vi "RT_SynthFoc_V2.vi"(0 "Ann Array Params":T1={"Synth Foc?"=FALSE, "Focal Zones"=41, "Switch T/R"=0, "Trans Geometry (mm)"={"Transducer"=0, "Geo Focus"=12.0, "a (radius)"=3.0, "# of rings"=5, "kerf space "=0.1, "Center Freq"=12.0}, "Sub Ap Excite?"=FALSE, "Full Array Scan?"=FALSE, "Xmt/Rcv"={"XMIT"=[TRUE, TRUE, TRUE, TRUE, TRUE], "RCV"=[TRUE, TRUE, TRUE, TRUE, TRUE]}, "PulseSpacing (us)"=0.0, "Xmit Ring"=0, "XMIT CHS"=0, "RCV CHS"=0, "GPU?"=FALSE, "Save TIFF?"=FALSE, "downfactor"=1, "RCV 1CH"=0} {"RCV 1CH" items=["All", "1", "2", "3", "4", "5"]; "Trans Geometry (mm)"."Transducer" items=["6D 12R 40 MHz"=0, "10D 31R 20 MHz"=1, "10D 23R 20 MHz"=2, "6D 23R 40 MHz"=3, "4.5D 10.7R 40 MHz"=4, "9D 23.5R 20 MHz"=5, "9D 25.8R 20MHz"=6, "Enter"=99]; "Switch T/R" min=1 max=5 step=1}, 2 "Pause?":bool, 3 "Motion Settings":T4={"No Motion?"=FALSE, "Motion System"=enum."NI 735x", "Motion Bd ID"=1, "Motion Profile"="SMAC1", "# Axis"=1, "Reverse Z axis?"=TRUE, "SMAC Axis"=0, "scan pair"=enum."y-(x) scan", "RT fps"=6.0, "Steps per mm"=[1000, 1000, 1000, 1000], "Motor Parameters"={"velocity ct/s"=[10000.0, 10000.0, 10000.0, 50000.0], "accel ct/s^2"=[50000.0, 50000.0, 50000.0, 200000.0]}, "One Way Scan"=FALSE, "Reverse One Way Scan"=FALSE, "Global Position (mm)"=[], "Plane"=0, "Distance between\nscan lines (um)"=0.0, "Distance between\nscan planes (um)"=0.0, "number of scan planes"=1, "Total steps in line"=0, "Xtra plane\ndistance  (um)"=100, "Xtra planes "=1, "Add Axis"=FALSE, "overshoot cts"=200, "BKPT Shift"=0, "Scan Start Time (ms)"=0, "ESP VISA"="GPIB::1::INSTR", "3rd Axis"=1, "GL Ref Out"=refnum, "Galil Address"=""} {"3rd Axis" items=["x", "y", "z", "w"]; "Xtra planes" min=1; "Xtra plane\ndistance  (um)" min=0; "Distance between\nscan planes (um)" format="%.2f"; "Distance between\nscan lines (um)" format="%.2f"; "SMAC Axis" items=["None"=0, "Axis 1"=1, "Axis 2"=2, "Axis 3"=3, "Axis 4"=4, "Axis 5"=5, "Axis 6"=6, "Axis 7"=7, "Axis 8"=8, "Vector Space 1"=17, "Vector Space 2"=18, "Vector Space 3"=19, "Vector Space 4"=20]; "Motion Bd ID" min=1 max=32 step=1}, 4 "Scan Axis":i32, 7 "Digitizer Settings":T8={"Digitizer delay (us) "=0.0, "rf points per line"=2048, "lines per plane"=128, "Samp Rate (Hz)"=100000000.0, "Additional dig delay (us)"=0.0, "Voltage Scale"=0.4, "Pre-Looks"=0, "Offset delay (us)"=0.0, "bits A/D"=8, "Avg Num"=1, "DigTimeOut"=5.0, "Rel Dig Delay"=0.0, "Dig Ch"=0, "LeCroyCluster"={"LeCroy Channels"=[TRUE, FALSE, FALSE, FALSE], "LC read pt offset"=0.0, "Sweep Avg"=FALSE}, "Main Digitizer"=enum."NI Digitizer", "Dig Config"=enum."Single channel", "Digitizer ID Cluster"={"Acqiris/Alazar/SP ID"=[], "NI Instr Handles"=[], "LeCroy VISA"="", "GaGe Handle"={"Handle"=0, "Sample size"=0, "Resolution"=0, "Offset"=0, "Channels"=0, "Boards"=0}, "ATS Ref"="ATS9350", "Acqiris Address"=["PCI::INSTR0"], "ADQRef"=refnum, "adq_cu_ptr"=refnum}, "Trigger Settings"={"Trig Source"=1, "Trig Coupling"=0, "Trig Slope"=0, "Level (mV)"=1500.0}, "Bulk Acq"=FALSE, "Bulk Start Indexes"=[], "Data Ref RF"=refnum, "NI ID/Channel"=[], "Total Dig CH"=1, "Xtra Ann Trig delay (us)"=10.0, "Fix Z Delay?"=FALSE, "One Way Transmission?"=FALSE, "Data Ref Log"=refnum} {"Trigger Settings"."Trig Slope" items=["Positive", "Negative"]; "Trigger Settings"."Level (mV)" format="%.2f"; "Trigger Settings"."Trig Coupling" items=["DC 1 MOhm", "AC 1 MOhm", "DC 50 Ohm", "AC 50 Ohm"]; "Trigger Settings"."Trig Source" items=["Chan 1", "External"]; "Rel Dig Delay" format="%.2f"; "DigTimeOut" format="%.2f"; "Avg Num" min=1; "Offset delay (us)" format="%.2f"; "Additional dig delay (us)" format="%.2f"; "Digitizer delay (us)" format="%.2f"}, 8 "Filter":T12, 9 "Qs and Notis":T13, 11 "Raw Name":string="raw") -> (16 "Bd ID Out":u8, 19 "error out":errorcluster)   [LabVIEW 2022 SP3]
uses:
  <vilib>/picture/picture.llb/imagedata.ctl
  ScanningControl/Digitizers/-DigitizerRoutines/DigitizerSettings.ctl
  ScanningControl/Digitizers/-DigitizerRoutines/Digitizer.ctl
  ScanningControl/Digitizers/-DigitizerRoutines/DigConfig.ctl
  ScanningControl/Digitizers/-DigitizerRoutines/DigitizerID.ctl
  C:/Windows/System32/ADQAPI_dotNet_helper.dll
  Windows/System32/ADQAPI_dotNet_helper.dll
  ScanningControl/Motion Controllers/NI_controller/-NI_MotionRoutines/MotionParameters.ctl
  ScanningControl/Motion Controllers/NI_controller/-NI_MotionRoutines/MotionSys.ctl
  ScanningControl/Motion Controllers/-MotionRoutines/ScanAxis.ctl
  ScanningControl/Motion Controllers/-MotionRoutines/3rdAxis.ctl
  Annular Array/-AnnularRoutines/AnnularArray.ctl
  Annular Array/-AnnularRoutines/TransGeometry.ctl
  Annular Array/-AnnularRoutines/ArrayGeometry.ctl
  ScanningControl/Motion Controllers/Galil/Command Menu.ctl
  <vilib>/DAQmx/write.llb/DAQmx Write (Digital Bool 1Line 1Point).vi
  <instrlib>/niScope/Acquire/niScope Get Scaling Coefficients.vi
  ScanningControl/Motion Controllers/-MotionRoutines/MotionGlobals.vi
  <vilib>/DAQmx/miscellaneous.llb/DAQmx Fill In Error Info.vi
  <instrlib>/niScope/Acquire/Fetch/niScope Multi Fetch Binary 8.vi
  <vilib>/Motion/FlexMotion/FunctionsVIs/Trajectory.llb/Load Acceleration/Deceleration.flx
  <vilib>/Motion/FlexMotion/CustomControls/CustomControls.llb/Program.flx
  <instrlib>/LeCroy Wave Series/LeCroy Wave Series.lvlib
  <vilib>/Motion/FlexMotion/FunctionsVIs/Trajectory.llb/Wait for Move Complete (8 axes).flx
panel:
  in  "Round to ROC?":bool
  in  "One Way Receive":bool
  # "1-D and 2-D B scan settings"
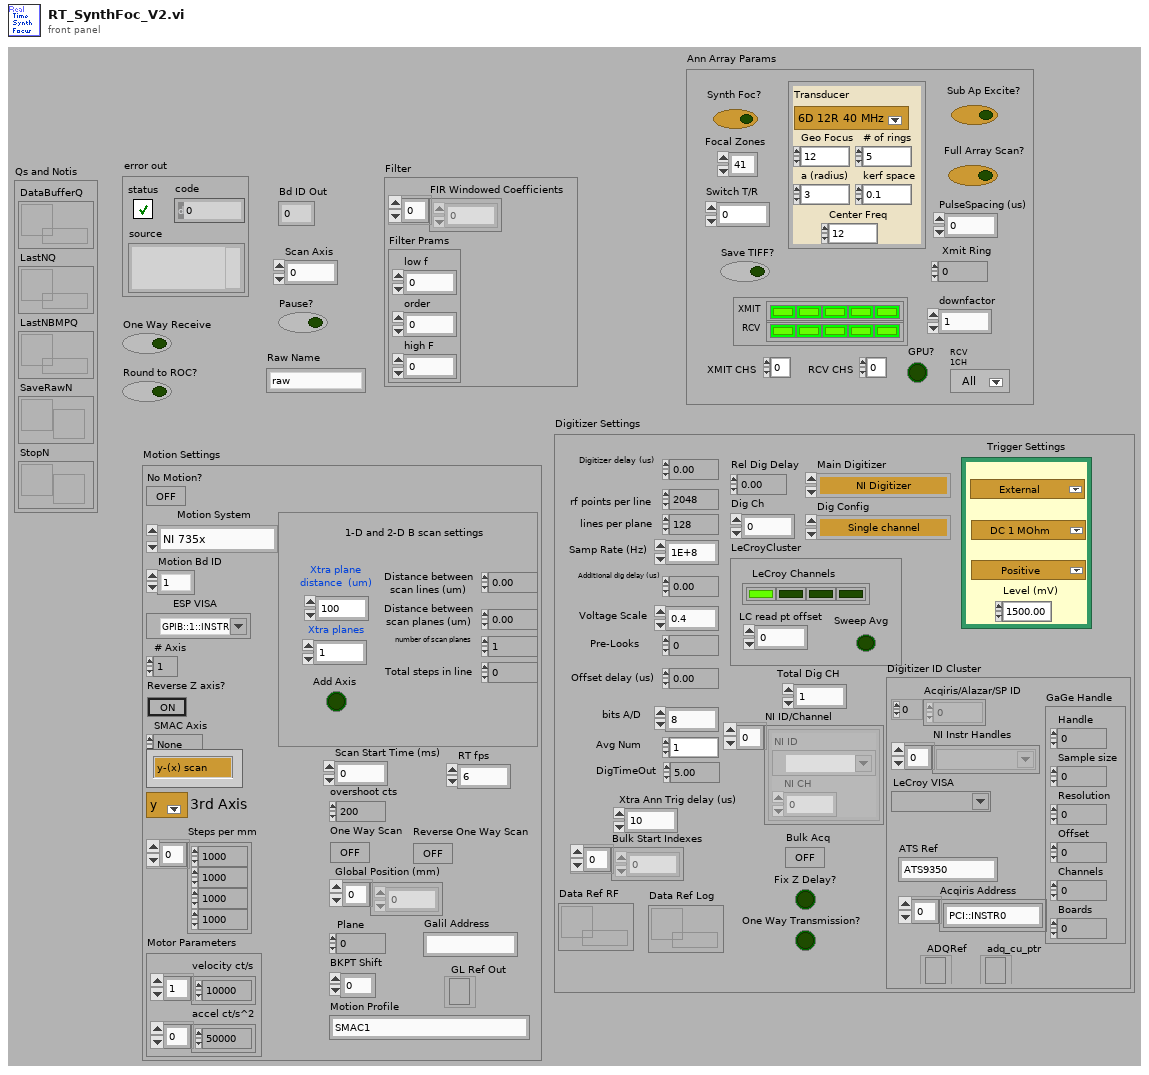
[diagram p1: front panel]
types:
  T1 = typedef "AnnularArray.ctl" = cluster{"Synth Foc?":bool, "Focal Zones":i16, "Switch T/R":i16, "Trans Geometry (mm)":T2, "Sub Ap Excite?":bool, "Full Array Scan?":bool, "Xmt/Rcv":cluster{"XMIT":bool[], "RCV":bool[]}, "PulseSpacing (us)":sgl, "Xmit Ring":i32, "XMIT CHS":u8, "RCV CHS":u8, "GPU?":bool, "Save TIFF?":bool, "downfactor":i32, "RCV 1CH":u16}
  T2 = typedef "TransGeometry.ctl" = cluster{"Transducer":T3, "Geo Focus":dbl, "a (radius)":dbl, "# of rings":i32, "kerf space ":dbl, "Center Freq":dbl}
  T3 = typedef "ArrayGeometry.ctl" = u16
  T4 = typedef "MotionParameters.ctl" = cluster{"No Motion?":bool, "Motion System":T5, "Motion Bd ID":u8, "Motion Profile":string, "# Axis":i8, "Reverse Z axis?":bool, "SMAC Axis":u16, "scan pair":T6, "RT fps":sgl, "Steps per mm":i32[], "Motor Parameters":cluster{"velocity ct/s":dbl[], "accel ct/s^2":dbl[]}, "One Way Scan":bool, "Reverse One Way Scan":bool, "Global Position (mm)":dbl[], "Plane":i32, "Distance between\nscan lines (um)":sgl, "Distance between\nscan planes (um)":sgl, "number of scan planes":i32, "Total steps in line":i32, "Xtra plane\ndistance  (um)":i32, "Xtra planes ":i32, "Add Axis":bool, "overshoot cts":i32, "BKPT Shift":i32, "Scan Start Time (ms)":u32, "ESP VISA":refnum<visa-resource-name>, "3rd Axis":T7, "GL Ref Out":refnum<k7>, "Galil Address":string}
  T5 = typedef "MotionSys.ctl" = enum16{"MM3000", "NI 735x", "Newport ESP", "No Motion Card", "Galil"}
  T6 = typedef "ScanAxis.ctl" = enum16{"y-(x) scan", "x-(y) scan", "z-(x) scan", "z-(y) scan", "y-(z) scan", "x-(z) scan", "w-(x) scan", "w-(y) scan", "w-(z) scan", "x-(w) scan", "y-(w) scan", "z-(w) scan"}
  T7 = typedef "3rdAxis.ctl" = u16
  T8 = typedef "DigitizerSettings.ctl" = cluster{"Digitizer delay (us) ":dbl, "rf points per line":i32, "lines per plane":i32, "Samp Rate (Hz)":dbl, "Additional dig delay (us)":dbl, "Voltage Scale":dbl, "Pre-Looks":i32, "Offset delay (us)":dbl, "bits A/D":i8, "Avg Num":i32, "DigTimeOut":sgl, "Rel Dig Delay":sgl, "Dig Ch":i32, "LeCroyCluster":cluster{"LeCroy Channels":bool[], "LC read pt offset":dbl, "Sweep Avg":bool}, "Main Digitizer":T9, "Dig Config":T10, "Digitizer ID Cluster":T11, "Trigger Settings":cluster{"Trig Source":u16, "Trig Coupling":u16, "Trig Slope":u16, "Level (mV)":dbl}, "Bulk Acq":bool, "Bulk Start Indexes":i32[], "Data Ref RF":refnum<data-value>, "NI ID/Channel":cluster{"NI ID":refnum<k15>, "NI CH":i32}[], "Total Dig CH":i32, "Xtra Ann Trig delay (us)":dbl, "Fix Z Delay?":bool, "One Way Transmission?":bool, "Data Ref Log":refnum<data-value>}
  T9 = typedef "Digitizer.ctl" = enum16{"Acqiris Digitizer", "NI Digitizer", "LeCroy", "GaGe", "AlazarTech", "No Digitizer", "Teledyne"}
  T10 = typedef "DigConfig.ctl" = enum16{"Single channel", "2 Chans w/ 2 Acqiris", "2 Chans w/ 1 Acqiris", "5-CH Pulser New", "5-CH pulser w/ ann array", "5-pass style ann array", "Empty"}
  T11 = typedef "DigitizerID.ctl" = cluster{"Acqiris/Alazar/SP ID":u32[], "NI Instr Handles":refnum<k15>[], "LeCroy VISA":refnum<visa-resource-name>, "GaGe Handle":cluster{"Handle":u32, "Sample size":u32, "Resolution":i32, "Offset":i32, "Channels":u32, "Boards":u32}, "ATS Ref":string, "Acqiris Address":string[], "ADQRef":refnum<k24>, "adq_cu_ptr":refnum<k24>}
  T12 = cluster{"FIR Windowed Coefficients":dbl[], "Filter Prams":cluster{"low f":i32, "order":i32, "high F":i32}}
  T13 = cluster{"DataBufferQ":refnum<queue>, "LastNQ":refnum<queue>, "LastNBMPQ":refnum<queue>, "SaveRawN":refnum<notifier>, "StopN":refnum<notifier>}
  T14 = cluster{"offset":dbl, "gain":dbl, "reserved 1":dbl, "reserved 2":dbl}[]
  T15 = cluster{"offset":dbl, "gain":dbl, "reserved 1":dbl, "reserved 2":dbl}
  T16 = cluster{sgl, "Gain [dB]  ":sgl, "Atten (dB)":sgl}
  T17 = typedef "location.ctl" = enum16{"Automatic", "WCM Main", "Hawaii", "Columbia MM3000", "Columbia  NI System", "NYU", "RRI 2", "UHI Allen", "CUMC RT", "Chiba", "Stony Brook", "WCM Microscopy", "WCM Aeoretch", "WCM Optics Lab", "WCM Main 2Axis", "WCM Rotation", "WCM SAM SMAC", "SERI GP"}
  T18 = typedef "Command Menu.ctl" = enum16{"CommandPassThrough", "Abort Motion", "Define Pos", "Velocity", "Acceleration", "Deceleration", "Position Rel", "Postion Abs", "Begin Move", "After Move", "Home", "KI", "KD", "KP", "IL", "Config I/O", "Set Bit", "Clear Bit", "Motor Off", "Moto On", "Status", "Execute", "Halt Execute", "HX Status", "Tell Velocity", "Check Motion", "BreakPoint", "Tell Position", "Current Code Line", "Tell Switches", "OC Force On", "OC Off", "Pos Soft Limit", "Rev Soft Limit"}
  T19 = cluster{"gain":dbl, "wfm":i16[][], bool, "max queue size (-1, unlimited)":i32, bool}
  T20 = typedef "Program.flx" = u8
  T21 = cluster{"Y Scale Offset":dbl, "Y Scale Multi":dbl, "X Scale Offset":dbl, "X Scale Multi":dbl, "Gate Distance":dbl}
  T22 = cluster{"ZoneStart":sgl[], "ZoneShift":sgl[], "ZoneLength":sgl[]}
  T23 = cluster{"data value reference":refnum<data-value>, "bytes to transfer":u32, "rf pts actual":u32}
  T24 = cluster{"gain":dbl, bool, i16[][], "Sat Pts":i32, bool}
  T25 = cluster{"actualSamples":i32, "absoluteInitialX":dbl, "relativeInitialX":dbl, "xIncrement":dbl, "offset":dbl, "gain":dbl, "reserved1":dbl, "reserved2":dbl}[]
  T26 = cluster{"actualSamples":i32, "absoluteInitialX":dbl, "relativeInitialX":dbl, "xIncrement":dbl, "offset":dbl, "gain":dbl, "reserved1":dbl, "reserved2":dbl}
  T27 = cluster{"gain":dbl, "wfm":i16[][], "Reverse?":bool, i32, "status":bool}
  T28 = cluster{"Voltage Scale":dbl, i16[][], "Reverse?":bool, i32, bool}
  T29 = cluster{"Raw VGain (scale)":dbl, i16[][], "Reverse?":bool, i32, "x = y?":bool}
  T30 = typedef "Bd Id Out" = u8
  T31 = typedef "Resource Out (Enum).flx" = u16
  T32 = typedef "GL Axis Control.ctl" = u16
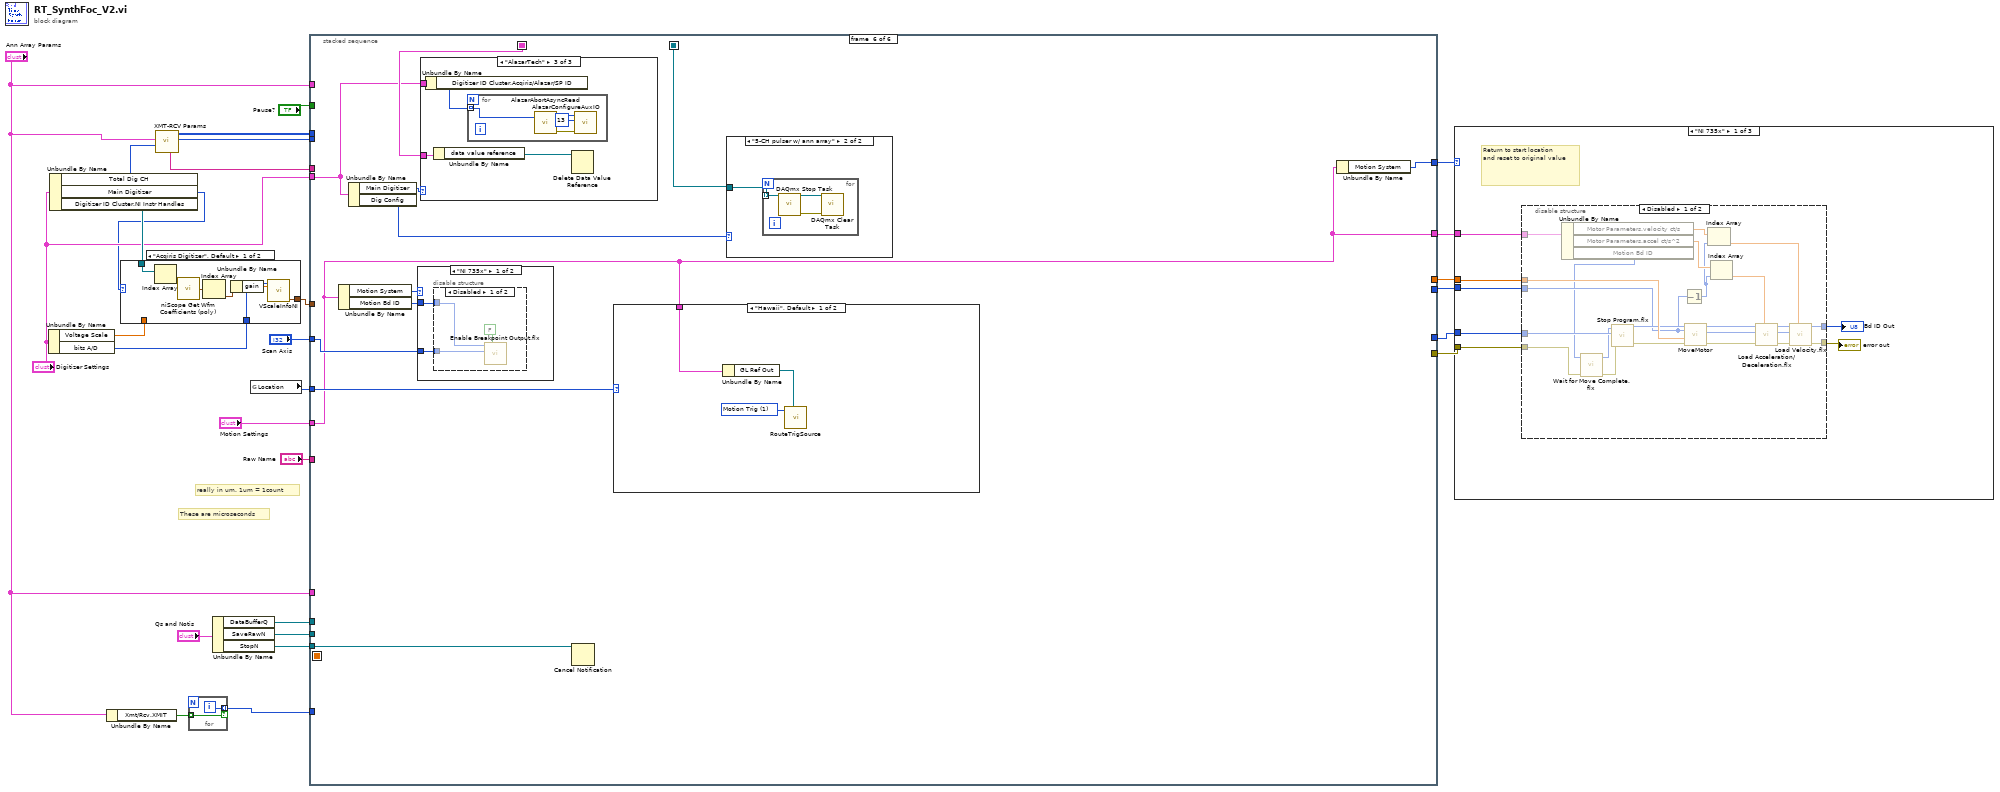
[diagram p0: block diagram]
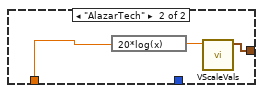
[diagram p2: hidden frame]
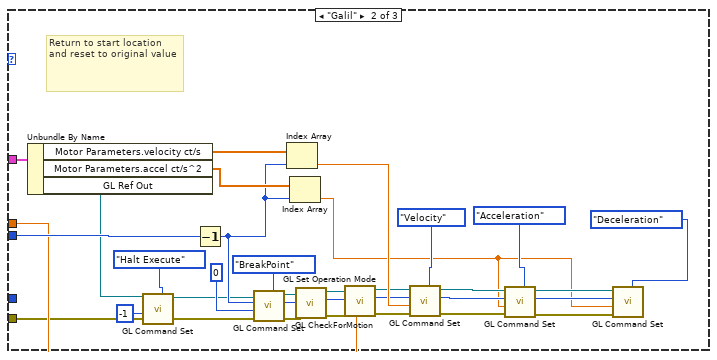
[diagram p4: hidden frame]
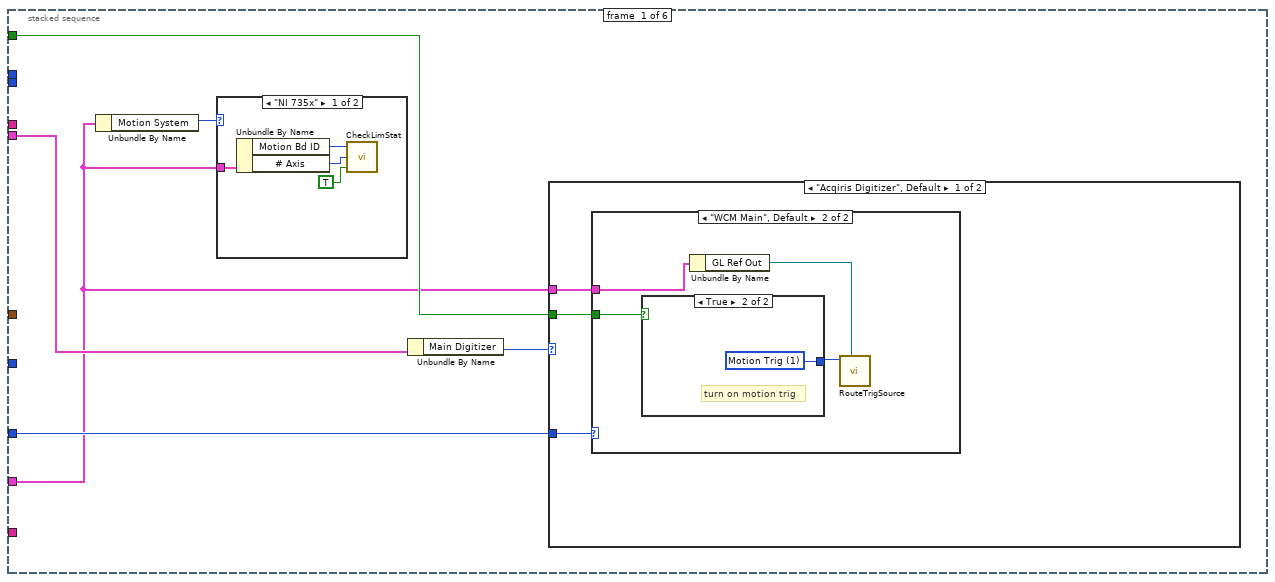
[diagram p6: hidden frame]
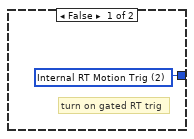
[diagram p8: hidden frame]
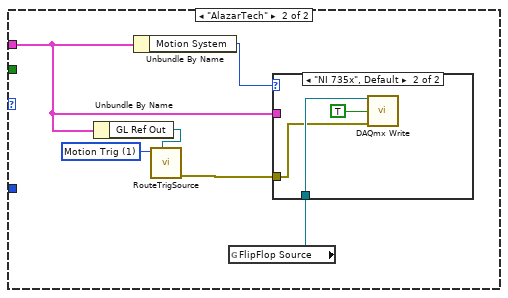
[diagram p9: hidden frame]
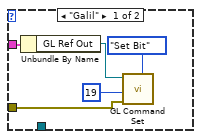
[diagram p10: hidden frame]
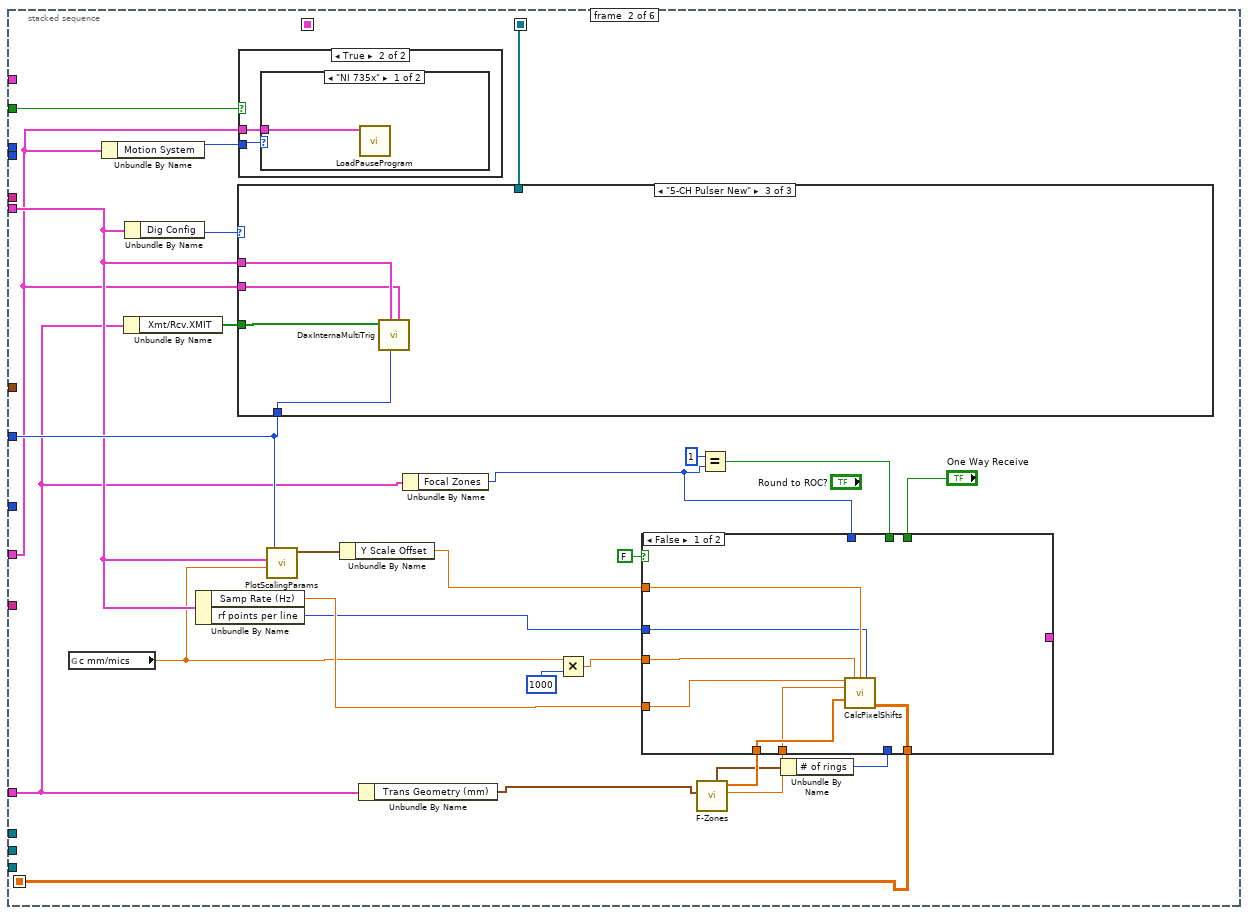
[diagram p12: hidden frame]
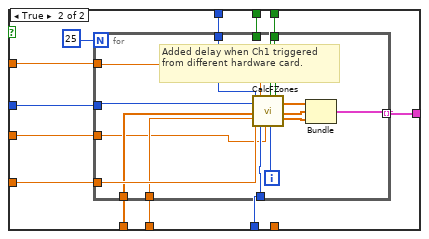
[diagram p13: hidden frame]
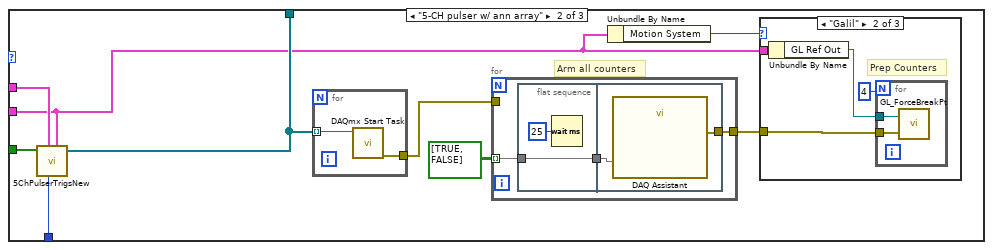
[diagram p15: hidden frame]
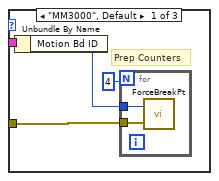
[diagram p16: hidden frame]
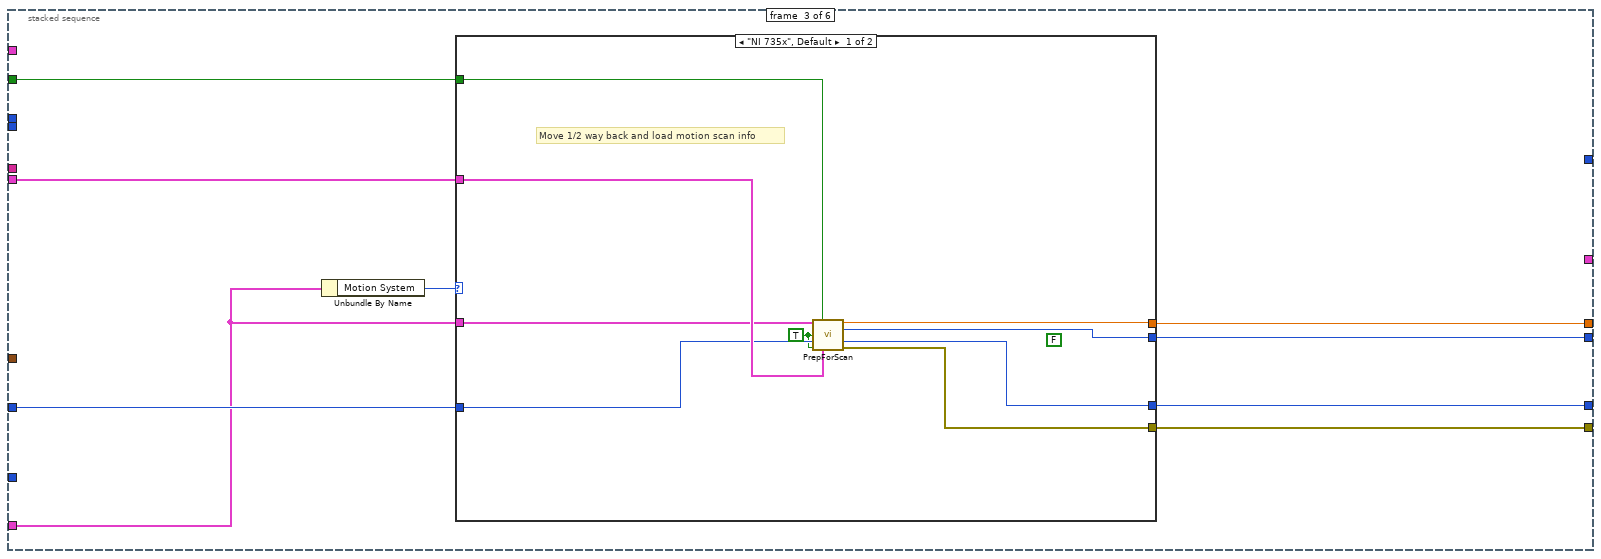
[diagram p20: hidden frame]
diagram:
  # "These are microseconds"
  # "really in um. 1um = 1count"
  n1 = Unbundle By Name("Digitizer Settings") -> ("Voltage Scale"=w13:dbl, "bits A/D"=w12:i8)
  n2 = Unbundle By Name("Digitizer Settings") -> ("Total Dig CH"=w4:i32, "Main Digitizer"=w10:T9, "Digitizer ID Cluster.NI Instr Handles"=w14:refnum<k15>[])
  n3 = Unbundle By Name("Ann Array Params") -> ("Xmt/Rcv.XMIT"=w3:bool[])
  n4 = case shown="\"Acqiris Digitizer\", Default" w10 {
    tunnel: [w31 w37] -> w17
    tunnel: w14 -> [w30 _]
    tunnel: w12 -> [w29 _]
    tunnel: w13 -> [_ w36]
    frame "Acqiris Digitizer", Default {
      n5 = Index Array(array=w30) -> (element=w33:refnum<k15>)  [unwired: 1 in]
      n6 = call-poly <instrlib>:"niScope Get Wfm Coefficients (poly).vi"("instrument handle"=w33) -> ("coefficient info"=w34:T14)  [unwired: 12 in, 2 out]
      n7 = Index Array(array=w34) -> (element=w35:T15)  [unwired: 1 in]
      n8 = Unbundle By Name(w35) -> ("gain"=w32:dbl)
      n9 = call "VScaleInfoNI.vi"("A/D bits"=w29, "gain"=w32) -> ("Voltage Scale"=w31:T16)  [unwired: 5 in, 3 out]
    }
    frame "AlazarTech" {
      n10 = expression code="20*log(x)"(w36) -> (w38:dbl)
      n11 = call "VScaleVals.vi"("Full Scale"=w38) -> ("Voltage Scale"=w37:T16)  [unwired: 8 in, 2 out]
    }
  }
  n12 = call "XMT-RCV Params.vi"("Dig Channels"=w4, "Ann Array Params"="Ann Array Params") -> ("# XMIT"=w16:i16, "Recip Table"=w15:i16[][], "T/R String"=w9:string)  [unwired: 4 in, 3 out]
  n13 = for {
    tunnel: w3 -> [w39] mode=indexing
    tunnel: [w40] -> w1 mode=indexing if=w39
    i -> [w40]
  }
  n14 = Unbundle By Name("Qs and Notis") -> ("DataBufferQ"=w22:refnum<queue>, "SaveRawN"=w21:refnum<notifier>, "StopN"=w23:refnum<notifier>)
  n15 = global read "MotionGlobals.vi" "Location"() -> (w18:T17)
  n16 = stacked-sequence {
    seq-local: [_ w74 _ _ _ _] -> [_ _ _ _ w248 _]
    seq-local: [_ w98 _ _ _ _] -> [_ _ _ _ _ w679]
    seq-local: [_ _ _ w195 _ _] -> [_ _ _ _ w260 w675]
    tunnel: [_ _ w180 _ _ _] -> w26
    tunnel: [_ _ w179 _ _ _] -> w27
    tunnel: [_ _ w176 _ _ _] -> w25
    tunnel: [_ _ w178 _ _ _] -> w28
    tunnel: "Scan Axis" -> [_ w91 w177 _ _ w676]
    tunnel: w23 -> [_ _ _ _ w289 w677]
    tunnel: w22 -> [_ _ _ _ w274 _]
    tunnel: w18 -> [w46 _ _ _ _ w678]
    tunnel: "Pause?" -> [w45 w99 w175 w190 w286 _]
    tunnel: w21 -> [_ _ _ _ w285 _]
    tunnel: "Raw Name" -> [_ _ _ _ w284 _]
    tunnel: w17 -> [_ _ _ _ w282 _]
    tunnel: w16 -> [_ _ _ w197 w280 _]
    tunnel: w15 -> [_ _ _ _ w255 _]
    tunnel: w9 -> [_ _ _ _ w279 _]
    tunnel: "Digitizer Settings" -> [w43 w87 w174 w192 w250 w674]
    tunnel: "Motion Settings" -> [w41 w79 w173 _ w265 w668]
    tunnel: [_ _ _ _ _ w669] -> w8
    tunnel: [_ _ _ _ _ w668] -> w7
    tunnel: "Ann Array Params" -> [_ w81 _ _ w252 _]
    tunnel: "Ann Array Params" -> [_ _ _ _ w254 _]
    tunnel: w1 -> [_ _ _ _ w249 _]
    frame #0 {
      n17 = Unbundle By Name(w41) -> ("Motion System"=w42:T5)
      n18 = case shown="\"NI 735x\"" w42 {
        tunnel: w41 -> [w73 _]
        frame "NI 735x" {
          n19 = Unbundle By Name(w73) -> ("Motion Bd ID"=w72:u8, "# Axis"=w71:i8)
          n20 = call "CheckLimStat.vi"("Always Warn?"=TRUE, "# Axis"=w71, "Motion Board ID"=w72) -> ()  [unwired: 3 in]
        }
        frame "Newport ESP", "No Motion Card", Default {
        }
      }
      n21 = Unbundle By Name(w43) -> ("Main Digitizer"=w44:T9)
      n22 = case shown="\"Acqiris Digitizer\", Default" w44 {
        tunnel: w46 -> [w49 _]
        tunnel: w45 -> [w48 _]
        tunnel: w41 -> [w47 w57]
        frame "Acqiris Digitizer", Default {
          n23 = case shown="\"WCM Main\", Default" w49 {
            tunnel: w48 -> [_ w53]
            tunnel: w47 -> [_ w51]
            frame "UHI Allen", "CUMC RT" {
            }
            frame "WCM Main", Default {
              n24 = case shown="True" w53 {
                tunnel: [w54 w55] -> w52
                frame False {
                  w54 = u16 2 items=["Function Gen Input", "Motion Trig", "Internal RT Motion Trig", "Internal CTR 1 Output"] ("Trig Source")
                  # "turn on gated RT trig"
                }
                frame True {
                  w55 = u16 1 items=["Function Gen Input", "Motion Trig", "Internal RT Motion Trig", "Internal CTR 1 Output"] ("Trig Source")
                  # "turn on motion trig"
                }
              }
              n25 = Unbundle By Name(w51) -> ("GL Ref Out"=w50:refnum<k7>)
              n26 = call "RouteTrigSource.vi"("Galil.IGalil"=w50, "Trig Source"=w52) -> ()  [unwired: 9 in, 1 out]
            }
          }
        }
        frame "AlazarTech" {
          w61 = u16 1 items=["Function Gen Input", "Motion Trig", "Internal RT Motion Trig", "Internal CTR 1 Output"] ("Trig Source")
          n27 = Unbundle By Name(w57) -> ("GL Ref Out"=w56:refnum<k7>)
          n28 = Unbundle By Name(w57) -> ("Motion System"=w59:T5)
          n29 = call "RouteTrigSource.vi"("Galil.IGalil"=w56, "Trig Source"=w61) -> ("error out"=w58:errorcluster)  [unwired: 9 in]
          n30 = global read "MotionGlobals.vi" "FlipFlop Source"() -> (w60:refnum<k21>)
          n31 = case shown="\"NI 735x\", Default" w59 {
            tunnel: w60 -> [_ w68]
            tunnel: w57 -> [w63 _]
            tunnel: w58 -> [w62 w67]
            frame "Galil" {
              n32 = Unbundle By Name(w63) -> ("GL Ref Out"=w66:refnum<k7>)
              n33 = call "GL Command Set.vi"("Command"=Command_Menu."Set Bit", "error in (no error)"=w62, "Value"=19, "Galil.IGalil"=w66) -> ()  [unwired: 3 in, 5 out]
            }
            frame "NI 735x", Default {
              n34 = call-poly <vilib>:"DAQmx Write.vi"("task/channels in"=w68, "data"=TRUE ("stop (T)"), "error in"=w67) -> ()  [unwired: 10 in, 3 out]
            }
          }
        }
      }
    }
    frame #1 {
      n35 = global read "MotionGlobals.vi" "c mm/mics"() -> (w77:sgl)
      n36 = Unbundle By Name(w79) -> ("Motion System"=w86:T5)
      n37 = Unbundle By Name(w81) -> ("Xmt/Rcv.XMIT"=w82:bool[])
      n38 = Unbundle By Name(w87) -> ("Dig Config"=w88:T10)
      n39 = Unbundle By Name(w87) -> ("Samp Rate (Hz)"=w93:dbl, "rf points per line"=w92:i32)
      n40 = case shown="\"5-CH Pulser New\"" w88 {
        tunnel: w91 -> [_ w143 w165]
        tunnel: [_ w142 _] -> w98
        tunnel: w82 -> [_ w138 w166]
        tunnel: w87 -> [_ w137 w168]
        tunnel: w79 -> [_ w135 w167]
        frame "Single channel", Default {
        }
        frame "5-CH pulser w/ ann array" {
          # "Arm all counters"
          n41 = call "5ChPulserTrigsNew.vi"("Motion Settings"=w135, "Digitizer Settings"=w137, "XMIT"=w138, "Axis"=w143) -> ("5CH Pulser Tasks"=w142:refnum<k21>[])  [unwired: 5 in, 1 out]
          n42 = for {
            tunnel: w142 -> [w157] mode=indexing
            tunnel: [w156] -> w140
            n43 = call <vilib>:"DAQmx Start Task.vi"("task/channels in"=w157) -> ("error out"=w156:errorcluster)  [unwired: 1 in, 13 out]
          }
          n44 = for {
            tunnel: bool[][] [[TRUE], [FALSE]] ("data") -> [w159] mode=indexing
            tunnel: w140 -> [_]
            tunnel: [w158] -> w139
            n45 = flat-sequence {
              tunnel: w159 -> [w162]
              tunnel: [w162] -> w160
              tunnel: w160 -> [w164]
              tunnel: [w163] -> w158
              frame #0 {
                n46 = Wait (ms)(milliseconds to wait=u32 25) -> ()  [unwired: 1 out]
              }
              frame #1 {
                n47 = call "DAQ Assistant"("data"=w164) -> ("error out"=w163:errorcluster)  [unwired: 17 in, 1 out]
              }
            }
          }
          n48 = Unbundle By Name(w135) -> ("Motion System"=w136:T5)
          n49 = case shown="\"Galil\"" w136 {
            tunnel: w139 -> [w146 w152 _]
            tunnel: w135 -> [w145 w150 _]
            frame "MM3000", Default {
              # "Prep Counters"
              n50 = Unbundle By Name(w145) -> ("Motion Bd ID"=w144:u8)
              n51 = for {
                N: 4 -> [_]
                tunnel: w144 -> [w149]
                tunnel: w146 -> [w148]
                n52 = call "ForceBreakPt.vi"("error in"=w148, "Bd ID in"=w149) -> ()  [unwired: 2 out]
              }
            }
            frame "Galil" {
              # "Prep Counters"
              n53 = Unbundle By Name(w150) -> ("GL Ref Out"=w151:refnum<k7>)
              n54 = for {
                N: 4 -> [_]
                tunnel: w151 -> [w155]
                tunnel: w152 -> [w154]
                n55 = call "GL_ForceBreakPt.vi"("error in"=w154, "GL Ref Out"=w155) -> ()  [unwired: 2 out]
              }
            }
            frame "No Motion Card" {
            }
          }
        }
        frame "5-CH Pulser New" {
          n56 = call "DaxInternaMultiTrig.vi"("Motion Settings"=w167, "Digitizer Settings"=w168, "XMIT"=w166, "Axis"=w165) -> ()  [unwired: 6 in, 1 out]
        }
      }
      n57 = case shown="True" w99 {
        tunnel: w86 -> [_ w170]
        tunnel: w79 -> [_ w169]
        frame False {
        }
        frame True {
          n58 = case shown="\"NI 735x\"" w170 {
            tunnel: w169 -> [w171 _]
            frame "NI 735x" {
              n59 = call "LoadPauseProgram.vi"("Motion Settings"=w171) -> ()  [unwired: 10 in, 1 out]
            }
            frame "No Motion Card", Default {
            }
          }
        }
      }
      n60 = call "PlotScalingParams.vi"("c mm/mics"=w77, "Digitizer Settings"=w87, "Scan Axis"=w91) -> ("Cluster"=w90:T21)  [unwired: 6 in, 2 out]
      n61 = Unbundle By Name(w90) -> ("Y Scale Offset"=w89:dbl)
      n62 = Unbundle By Name(w81) -> ("Trans Geometry (mm)"=w83:T2)
      n63 = Unbundle By Name(w81) -> ("Focal Zones"=w80:i16)
      n64 = Multiply(x=w77, y=1000) -> (x*y=w76:sgl)
      n65 = call "F-Zones.vi"("Trans Geometry (mm)"=w83) -> ("ROC (m)"=w96:dbl, "annuli rad (m)"=w97:dbl[], "Trans Geometry (mm) out"=w85:T2)  [unwired: 7 in, 1 out]
      n66 = Equal?(x=i16 1, y=w80) -> (x = y?=w94:bool)
      n67 = Unbundle By Name(w85) -> ("# of rings"=w84:i32)
      n68 = case shown="False" FALSE {
        tunnel: "One Way Receive" -> [_ w119]
        tunnel: w97 -> [w106 w117]
        tunnel: w96 -> [w105 w116]
        tunnel: [_ w115] -> _
        tunnel: w94 -> [_ w114]
        tunnel: w93 -> [w107 w113]
        tunnel: w92 -> [w102 w112]
        tunnel: w89 -> [w103 w111]
        tunnel: w76 -> [w104 w110]
        tunnel: w84 -> [_ w109]
        tunnel: w80 -> [_ w108]
        tunnel: [w101 _] -> w74
        frame False {
          n69 = call "CalcPixelShifts.vi"("Sampling Rate (Hz)"=w107, "c (m/s)"=w104, "delay (mm)"=w103, "rf pts"=w102, "ROC (m)"=w105, "Radii (m)"=w106) -> ("InterpIndex"=w101:sgl[][])  [unwired: 9 in]
        }
        frame True {
          n70 = for {
            N: 25 -> [_]
            tunnel: w112 -> [w134]
            tunnel: w110 -> [w120]
            tunnel: w113 -> [w129]
            tunnel: w111 -> [w122]
            tunnel: w119 -> [w133]
            tunnel: w114 -> [w132]
            tunnel: [w130] -> w115 mode=indexing
            tunnel: w117 -> [w126]
            tunnel: w116 -> [w125]
            tunnel: w108 -> [w123]
            tunnel: w109 -> [w121]
            i -> [w124]
            # "Added delay when Ch1 triggered from different hardware card."
            n71 = call "CalcFZones.vi"("F- zones"=w123, "# rf points per line"=w134, "Radii (m)"=w126, "ROC (m)"=w125, "Sampling Rate"=w129, "delay (mm)"=w122, "# Elements"=w121, "c (m/s)"=w120, "Round to ROC?"=w132, "File index number"=w124, "One Way Receive"=w133) -> ("ZoneStart"=w128:sgl[], "ZoneShift"=w127:sgl[], "ZoneLength"=w131:sgl[])  [unwired: 3 in, 3 out]
            n72 = Bundle("ZoneStart"=w128, "ZoneShift"=w127, "ZoneLength"=w131) -> (w130:T22)  [unwired: 1 in]
          }
        }
      }
    }
    frame #2 {
      n73 = Unbundle By Name(w173) -> ("Motion System"=w172:T5)
      n74 = case shown="\"NI 735x\", Default" w172 {
        tunnel: [w186 _] -> w180
        tunnel: [w185 _] -> w179
        tunnel: [w184 _] -> w178
        tunnel: w177 -> [w188 _]
        tunnel: [w187 _] -> w176
        tunnel: w175 -> [w182 _]
        tunnel: w174 -> [w189 _]
        tunnel: w173 -> [w181 _]
        frame "NI 735x", Default {
          w183 = TRUE ("Boolean")
          (unwired) FALSE ("Enable")
          # "Move 1/2 way back and load motion scan info"
          n75 = call "PrepForScan.vi"("Motion Settings In"=w181, "Pause?"=w182, "SMAC?"=w183, "Scan Axis"=w188, "MoveBack?"=w183, "Digitizer Settings"=w189) -> ("Counts"=w187:dbl, "Axis Resource out"=w184:u16, "Program ID"=w185:u8, "error out"=w186:errorcluster)  [unwired: 4 in, 2 out]
        }
        frame "No Motion Card" {
        }
      }
    }
    frame #3 {
      # "Set up sampling rete and delay"
      n76 = Unbundle By Name(w192) -> ("Main Digitizer"=w191:T9, "lines per plane"=w193:i32, "rf points per line"=w194:i32)
      n77 = Multiply(x=w197, y=w193) -> (x*y=w196:i32)
      n78 = case shown="\"AlazarTech\"" w191 {
        tunnel: w194 -> [w201 w214 _]
        tunnel: w196 -> [w200 w215 w230]
        tunnel: [_ w218 _] -> w195
        tunnel: w192 -> [w198 w216 w233]
        tunnel: w190 -> [_ w209 _]
        frame "Acqiris Digitizer", Default {
          n79 = Unbundle By Name(w198) -> ("Digitizer ID Cluster.NI Instr Handles"=w199:refnum<k15>[])
          n80 = for {
            tunnel: w200 -> [w204]
            tunnel: w201 -> [w208]
            tunnel: w199 -> [w205] mode=indexing
            tunnel: w198 -> [w202]
            n81 = property class="niScope"(reference=w205, "Min Number of Points"=w208, "Number of Records"=w204, "Enable Records > Memory"=TRUE) -> (reference out=w207:refnum<k15>, error out=w206:errorcluster)  [unwired: 1 in]
            n82 = call "NI conSamp.vi"("error in"=w206, "Digitizer Settings"=w202, "InstrumentID"=w207) -> ()  [unwired: 1 in, 2 out]
          }
        }
        frame "AlazarTech" {
          n83 = Unbundle By Name(w216) -> ("Digitizer ID Cluster.Acqiris/Alazar/SP ID"=w212:u32[], "Digitizer ID Cluster.GaGe Handle.Boards"=w210:u32)
          n84 = case shown="2, Default" w210 {
            tunnel: [w219 w220] -> w211
            frame 2, Default {
              w219 = u32 3 items=["A"=1, "B"=2, "A + B"=3, "C"=4, "A + C"=5, "A + B"=6, "D"=8, "A + D"=9, "B + D"=10, "C + D"=12, "A + B + C + D"=15] ("Channel")
            }
            frame 16 {
              w220 = u32 15 items=["A"=1, "B"=2, "A + B"=3, "C"=4, "A + C"=5, "A + B"=6, "D"=8, "A + D"=9, "B + D"=10, "C + D"=12, "A + B + C + D"=15] ("Channel")
            }
          }
          n85 = for {
            tunnel: [w229] -> w218
            tunnel: [w228] -> w217
            tunnel: w216 -> [w227]
            tunnel: w215 -> [w226]
            tunnel: w214 -> [w225]
            tunnel: w212 -> [w223] mode=indexing
            tunnel: w211 -> [w222]
            tunnel: w209 -> [w221]
            (unwired) TRUE ("Enable Trigger Enable")
            n86 = call "AlazarAcqPrep - ATS-SDK.vi"("Handle"=w223, "Digitizer Settings"=w227, "Enable Trigger Enable"=w221, "Channel"=w222, "BuffCount"=4, "rf points per line"=w225, "rf lines per buffer"=w226) -> ("AlazarCluster"=w229:T23, "error out"=w228:errorcluster)  [unwired: 5 in, 2 out]
          }
          n87 = Index Array(array=w212) -> (element=w213:u32)  [unwired: 1 in]
          n88 = call "AlazarStartCapture.vi"("Handle"=w213, "error in (no error)"=w217) -> ()  [unwired: 3 out]
        }
        frame "LeCroy" {
          w241 = FALSE ("Continuous Acquisition Mode (T: On)")
          w231 = u16 2 items=["RealTime", "RIS", "Sequence", "Roll", "WaveStream"] ("Sample Mode (0: RealTime)")
          n89 = Unbundle By Name(w233) -> ("Digitizer ID Cluster.LeCroy VISA"=w234:refnum<visa-resource-name>, "Digitizer delay (us)"=w232:dbl)
          n90 = call <instrlib>:"Configure Continuous Acquisition.vi"("Auto Trigger Enabled (T: Normal)"=w241, "Continuous Acquisition Mode (T: On)"=w241, "VISA resource name"=w234) -> ("error out"=w242:errorcluster, "VISA resource name out"=w243:refnum<visa-resource-name>)  [unwired: 7 in]
          n91 = expression code="-1E-6*x"(w232) -> (w239:dbl)
          n92 = call <instrlib>:"Configure Sample Mode.vi"("error in (no error)"=w242, "Number of Segments (2)"=w230, "Sample Mode (0: RealTime)"=w231, "VISA resource name"=w243) -> ("error out"=w237:errorcluster, "VISA resource name out"=w238:refnum<visa-resource-name>)  [unwired: 6 in]
          n93 = Number To Exponential String(number=w239) -> (E-format string=w240:string)  [unwired: 3 in]
          n94 = Concatenate Strings("TRDL " ("Write Buffer"), w240) -> (w236:string)
          n95 = call <instrlib>:"Write.vi"("error in (no error)"=w237, "Write Buffer"=w236, "VISA resource name"=w238) -> ()  [unwired: 6 in, 3 out]
        }
      }
    }
    frame #4 {
      w261 = i16 0
      n96 = Unbundle By Name(w250) -> ("bits A/D"=w266:i8, "lines per plane"=w267:i32, "rf points per line"=w268:i32, "Total Dig CH"=w244:i32)
      n97 = Unbundle By Name(w250) -> ("Total Dig CH"=w264:i32)
      n98 = Array Size(array=w248) -> (size(s)=w247:i32[])
      n99 = Index Array(array=w247, index=1) -> (element=w245:i32)
      n100 = Multiply(x=w264, y=3) -> (x*y=w263:i32)
      n101 = Initialize Array(i16 0, w267, w268) -> (w273:i16[][])
      n102 = Reshape Array(w248, w244, w244, w245) -> (w256:sgl[][][])
      n103 = New Data Value Reference(data value=w273) -> (data value reference=w287:refnum<data-value>)  [unwired: 1 in, 1 out]
      n104 = Unbundle By Name(w260) -> ("rf pts actual"=w259:u32)
      n105 = Multiply(x=w280, y=w267) -> (x*y=w258:i32)
      n106 = Unbundle By Name(w254) -> ("Xmt/Rcv.RCV"=w253:bool[])
      n107 = call "RTHeader.vi"("Comment"=w279, "Digitizer Settings"=w250, "Dig Word Size"=w266, "Ann Array Params"=w252, "Votage scaling"=w282, "Motion Settings"=w265) -> ("Header String Out"=w276:string)  [unwired: 8 in, 1 out]
      n108 = Obtain Queue(max queue size (-1, unlimited)=w263, element data type=T19 {"gain"=0.0, "wfm"=[], TRUE, "max queue size (-1, unlimited)"=12, TRUE}) -> (queue out=w275:refnum<queue>)  [unwired: 3 in, 2 out]
      n109 = case shown="14" w266 {
        tunnel: [_ u16 3 ("Extra Shift")] -> w269
        frame 0, Default {
        }
        frame 14 {
        }
      }
      n110 = Initialize Array(w261, w258, w259) -> (w257:i16[][])
      n111 = Initialize Array(w261, w258, w268) -> (w272:i16[][])
      n112 = Subtract(x=w266, y=w269) -> (x-y=w270:u16)
      n113 = while {
        tunnel: w275 -> [w323]
        tunnel: w268 -> [w322]
        tunnel: [w314] -> w271
        tunnel: w267 -> [w321]
        tunnel: w287 -> [w318]
        tunnel: w274 -> [w320]
        tunnel: [w312] -> w277
        tunnel: w276 -> [w316]
        tunnel: w289 -> [w293]
        tunnel: w285 -> [w311]
        tunnel: w284 -> [w310]
        tunnel: "Filter" -> [w305]
        tunnel: w280 -> [w304]
        tunnel: w255 -> [w303]
        tunnel: w256 -> [w302]
        tunnel: w253 -> [w297]
        tunnel: w270 -> [w296]
        tunnel: 1000 ("timeout in ms (-1)") -> [w292]
        tunnel: w249 -> [w291]
        i -> [w309]
        stop <- w314 stop-if-true
        n114 = for {
          tunnel: w322 -> [w344]
          tunnel: w321 -> [w347]
          tunnel: w323 -> [w326]
          tunnel: [w336] -> w306 mode=indexing
          tunnel: [w343] -> w319 mode=indexing
          tunnel: [w341] -> w317
          tunnel: w318 -> [w346]
          tunnel: w302 -> [w345]
          tunnel: w316 -> [w342]
          tunnel: w311 -> [w340]
          tunnel: w310 -> [w339]
          tunnel: w309 -> [w338]
          tunnel: [w337] -> w308 mode=indexing
          tunnel: w305 -> [w335]
          tunnel: w304 -> [w334]
          tunnel: w303 -> [w333]
          tunnel: w297 -> [w331] mode=indexing
          tunnel: w296 -> [w332]
          tunnel: [w328] -> w295
          tunnel: [w327] -> w294
          tunnel: w293 -> [w327]
          tunnel: w292 -> [w325]
          tunnel: w291 -> [w324]
          n115 = Dequeue Element(queue=w326, timeout in ms (-1)=w325) -> (element=w329:T19)  [unwired: 1 in, 3 out]
          n116 = Unbundle(w329) -> (w328:bool)  [unwired: 4 out]
          n117 = Compound Arithmetic op=AND(w331, invert w328) -> (w330:bool)
          n118 = case shown="True" w330 {
            tunnel: w347 -> [_ w372]
            tunnel: w346 -> [w348 w371]
            tunnel: w345 -> [_ w369]
            tunnel: w344 -> [_ w367]
            tunnel: [_ w366] -> w343
            tunnel: w342 -> [_ w364]
            tunnel: [w348 w363] -> w341
            tunnel: w329 -> [_ w362]
            tunnel: w340 -> [_ w360]
            tunnel: w339 -> [_ w359]
            tunnel: w338 -> [_ w358]
            tunnel: [_ w357] -> w337
            tunnel: [_ w356] -> w336
            tunnel: w335 -> [_ w355]
            tunnel: w334 -> [_ w354]
            tunnel: w333 -> [_ w353]
            tunnel: w332 -> [_ w350]
            tunnel: w324 -> [_ w349]
            frame False {
            }
            frame True {
              n119 = Unbundle(w362) -> ("gain"=w366:dbl, "wfm"=w365:i16[][], w356:bool, "max queue size (-1, unlimited)"=w351:i32)  [unwired: 1 out]
              n120 = Index Array(array=w369, index (dim 1)=w351) -> (element=w368:sgl[][])  [unwired: 2 in]
              n121 = Index Array(array=w353, index (col)=w351) -> (element=w352:i16[])  [unwired: 1 in]
              n122 = Multiply(x=w367, y=w354) -> (x*y=w370:i32)
              n123 = Reshape Array(w365, w372, w370) -> (w373:i16[][])
              n124 = Get Notifier Status(notifier=w360) -> (current notification=w361:bool)  [unwired: 1 in, 4 out]
              n125 = for {
                tunnel: w368 -> [w381]
                tunnel: [w394] -> w363
                tunnel: w371 -> [w393]
                shift-right: [w389] -> _
                shift-left: w373 -> [w395]
                tunnel: w367 -> [w391]
                tunnel: [w387] -> w357 mode=indexing
                tunnel: w355 -> [w386]
                tunnel: w352 -> [w384]
                tunnel: w350 -> [w385]
                tunnel: w349 -> [w382] mode=indexing
                n126 = Index Array(array=w384, index=w382) -> (element=w383:i16)
                n127 = Index Array(array=w381, index (row)=w382) -> (element=w380:sgl[])  [unwired: 1 in]
                n128 = Delete From Array(array=w395, length=w391, index (col)=0 ("disabled index (col)")) -> (deleted portion=w390:i16[][], array with subset deleted=w389:i16[][])  [unwired: 1 in]
                n129 = call "TimeShiftDataSubMean.vi"("ZoneLength"=w380, "bits A/D"=w385, "Filter"=w386, "Array In"=w390) -> ("Sat Pts"=w387:i32, "Array Out"=w388:i16[][])  [unwired: 4 in]
                n130 = in-place {
                  in-place-border: w388 -> [w397]
                  in-place-border: w383 -> [w398]
                  n131 = in-place-dvr #1(w393) -> (w399:i16[][])  [unwired: 1 out]
                  n132 = case shown="2" w398 {
                    selector: w398 -> [_ w402]
                    tunnel: w397 -> [w401 w404]
                    tunnel: [w401 w403] -> w396
                    frame 1, Default {
                    }
                    frame 2 {
                      n133 = Multiply(x=w402, y=w404) -> (x*y=w403:i16[][])
                    }
                  }
                  n134 = Add(x=w396, y=w399) -> (x+y=w400:i16[][])
                  n135 = in-place-dvr #1(w400) -> (w394:refnum<data-value>)  [unwired: 1 out]
                }
              }
              n136 = case shown="True" w361 {
                tunnel: w351 -> [_ w378]
                tunnel: w365 -> [_ w375]
                tunnel: w364 -> [_ w379]
                tunnel: w359 -> [_ w377]
                tunnel: w358 -> [_ w376]
                tunnel: w356 -> [_ _]
                tunnel: w350 -> [_ w374]
                frame False {
                }
                frame True {
                  n137 = call "RawRT_Capture.vi"("A/D bits"=w374, "Raw data"=w375, "File Name In"=w377, "DigCard"=w378, "header"=w379, "Iter"=w376) -> ()  [unwired: 6 in]
                }
              }
            }
          }
        }
        n138 = Wait on Notification(notifier=w294, timeout in ms (-1)=5) -> (timed out?=w315:bool)  [unwired: 2 in, 3 out]
        n139 = Add Array Elements(numeric array=w308) -> (sum=w307:i32)
        n140 = Search 1D Array(1D array=w297, element=TRUE) -> (index of element=w298:i32)  [unwired: 1 in]
        n141 = Not(x=w315) -> (.not. x?=w314:bool)
        n142 = Index Array(array=w319, index=w298) -> (element=w300:dbl)
        n143 = Index Array(array=w306, index=w298) -> (element=w301:bool)
        n144 = in-place {
          in-place-border: w320 -> [w413]
          in-place-border: w301 -> [w412]
          in-place-border: w300 -> [w411]
          in-place-border: w307 -> [w407]
          in-place-border: w295 -> [w406]
          n145 = in-place-dvr #2(w317) -> (w408:i16[][])  [unwired: 1 out]
          n146 = Bundle("gain"=w411, w412, w408, "Sat Pts"=w407, w406) -> (w405:T24)  [unwired: 1 in]
          n147 = Multiply(x=i16 0, y=w408) -> (x*y=w410:i16[][])
          n148 = Lossy Enqueue Element(queue=w413, element=w405) -> ()  [unwired: 1 in, 4 out]
          n149 = in-place-dvr #2(w410) -> (w312:refnum<data-value>)  [unwired: 1 out]
        }
      }
      n150 = while {
        tunnel: w275 -> [w429]
        tunnel: w268 -> [w428]
        tunnel: [w427] -> w278
        tunnel: w289 -> [w419]
        tunnel: w286 -> [w426]
        tunnel: w253 -> [w425]
        tunnel: w272 -> [w424]
        tunnel: w260 -> [w423]
        tunnel: w258 -> [w422]
        tunnel: w250 -> [w414]
        tunnel: w269 -> [w420]
        tunnel: w265 -> [w417]
        tunnel: w257 -> [w416]
        i -> [w421]
        stop <- w418 stop-if-true
        # "Read queue and send to files. About same as reading channel by channel"
        n151 = Unbundle By Name(w414) -> ("Main Digitizer"=w415:T9)
        n152 = stacked-sequence {
          seq-local: [w435 _ _ _ _] -> [_ w481 _ _ _]
          seq-local: [_ w475 _ _ _] -> [_ _ _ w613 _]
          tunnel: w429 -> [_ w484 _ _ _]
          tunnel: w428 -> [_ w483 _ _ _]
          tunnel: [_ w482 _ _ _] -> w427
          tunnel: w426 -> [w436 _ _ _ _]
          tunnel: w425 -> [_ w480 _ _ _]
          tunnel: w415 -> [w434 w479 _ w614 _]
          tunnel: w424 -> [_ w478 _ _ _]
          tunnel: w423 -> [_ w477 _ w612 _]
          tunnel: w422 -> [w433 w476 _ _ _]
          tunnel: w421 -> [w432 _ _ _ _]
          tunnel: w414 -> [w430 w472 _ w611 _]
          tunnel: w420 -> [_ w474 _ _ _]
          tunnel: w419 -> [_ _ w608 _ _]
          tunnel: [_ _ w607 _ _] -> w418
          tunnel: w417 -> [w431 _ _ _ w648]
          tunnel: w416 -> [_ w473 _ _ _]
          frame #0 {
            # "Arm boards"
            n153 = case shown="\"AlazarTech\"" w434 {
              tunnel: w436 -> [w443 w461 w469]
              tunnel: [w442 w463 w470] -> w435
              tunnel: w433 -> [w441 _ w471]
              tunnel: w432 -> [_ _ _]
              tunnel: w430 -> [w440 w465 w467]
              tunnel: w431 -> [w437 w460 w468]
              frame "Acqiris Digitizer", Default {
                n154 = Unbundle By Name(w440) -> ("Digitizer ID Cluster.NI Instr Handles"=w439:refnum<k15>[])
                n155 = Reverse 1D Array(array=w439) -> (reversed array=w438:refnum<k15>[])
                n156 = for {
                  N -> [w448]
                  tunnel: w443 -> [w451]
                  tunnel: [w447] -> w442
                  tunnel: w441 -> [w446]
                  tunnel: w438 -> [w445] mode=indexing
                  tunnel: w437 -> [w444]
                  i -> [w449]
                  n157 = Subtract(x=w448, y=w449) -> (x-y=w450:i32)
                  n158 = case shown="1" w450 {
                    tunnel: [_ w459] -> w447
                    tunnel: w451 -> [_ w458]
                    tunnel: [w452 w457] -> _
                    tunnel: w445 -> [w453 w456]
                    tunnel: w446 -> [_ w455]
                    tunnel: w444 -> [_ w454]
                    frame 0, Default {
                      n159 = call <instrlib>:"niScope Initiate Acquisition.vi"("instrument handle"=w453) -> ("error out"=w452:errorcluster)  [unwired: 2 in, 12 out]
                    }
                    frame 1 {
                      # "Start Move"
                      n160 = call "Rapid Read_NI_Done.vi"("NI Card"=w456, "Motion Settings In"=w454, "records"=w455, "Pause?"=w458) -> ("Reverse?"=w459:bool, "error out"=w457:errorcluster)  [unwired: 10 in]
                    }
                  }
                }
              }
              frame "AlazarTech" {
                n161 = Unbundle By Name(w465) -> ("Digitizer ID Cluster.Acqiris/Alazar/SP ID"=w464:u32[])
                n162 = Index Array(array=w464) -> (element=w462:u32)  [unwired: 1 in]
                n163 = call "Rapid Read_Alazar_Done - ATS-SDK.vi"("Handle"=w462, "Motion Settings"=w460, "Pause?"=w461) -> ("Reverse?"=w463:bool)  [unwired: 10 in, 2 out]
              }
              frame "LeCroy" {
                n164 = Unbundle By Name(w467) -> ("Digitizer ID Cluster.LeCroy VISA"=w466:refnum<visa-resource-name>)
                n165 = call "Rapid Read_LeCroy_Done.vi"("Digitizer ID Cluster.LeCroy VISA"=w466, "Motion Settings In"=w468, "records"=w471, "Pause?"=w469) -> ("Reverse?"=w470:bool)  [unwired: 10 in, 1 out]
              }
            }
          }
          frame #1 {
            # "Read data"
            n166 = case shown="\"AlazarTech\"" w479 {
              tunnel: w484 -> [w493 w553 w584]
              tunnel: w483 -> [w492 w550 w581]
              tunnel: [w491 w552 w583] -> w482
              tunnel: w481 -> [w490 w551 w582]
              tunnel: w480 -> [w489 _ w573]
              tunnel: w478 -> [w488 _ _]
              tunnel: w477 -> [_ w544 _]
              tunnel: w476 -> [w487 w543 w580]
              tunnel: w472 -> [w486 w540 w579]
              tunnel: [_ w541 _] -> w475
              tunnel: w474 -> [_ w545 _]
              tunnel: w473 -> [_ w547 w575]
              frame "Acqiris Digitizer", Default {
                n167 = Unbundle By Name(w486) -> ("NI ID/Channel"=w485:cluster{"NI ID":refnum<k15>, "NI CH":i32}[])
                n168 = for {
                  tunnel: w492 -> [w508]
                  tunnel: w493 -> [w504]
                  tunnel: [w505] -> w491
                  tunnel: w490 -> [w502]
                  tunnel: w489 -> [w501] mode=indexing
                  tunnel: w487 -> [w499]
                  tunnel: w488 -> [w498]
                  tunnel: w485 -> [w496] mode=indexing
                  i -> [w500]
                  n169 = case shown="True" w501 {
                    tunnel: w508 -> [_ w532]
                    tunnel: [_ w531] -> w507
                    tunnel: [_ w525] -> w506
                    tunnel: w500 -> [_ w523]
                    tunnel: [_ w519] -> w495
                    tunnel: w499 -> [_ w517]
                    tunnel: w498 -> [_ w516]
                    tunnel: [FALSE ("status") w514] -> w497
                    tunnel: w496 -> [_ w512]
                    frame False {
                    }
                    frame True {
                      n170 = Unbundle By Name(w512) -> ("NI CH"=w511:i32, "NI ID"=w513:refnum<k15>)
                      n171 = Equal To 0?(x=w523) -> (x = 0?=w522:bool)
                      n172 = property class="niScope"(reference=w513, "Fetch Record Number"=0, "Fetch Number of Records"=w517) -> (reference out=w527:refnum<k15>, error out=w526:errorcluster)  [unwired: 1 in]
                      n173 = Number To Decimal String(number=w511) -> (decimal integer string=w510:string)  [unwired: 1 in]
                      n174 = Select(t=1.0, s=w522, f=0.5) -> (s? t:f=w519:dbl)
                      n175 = call-poly <instrlib>:"niScope Fetch (poly).vi"("timeout"=w519, "error in"=w526, "numSamples"=w532, "channels"=w510, "instrument handle"=w527) -> ("error out"=w515:errorcluster, "wfm"=w524:i8[][], "wfm info"=w530:T25, "instrument handle out"=w518:refnum<k15>)  [unwired: 3 out]
                      n176 = case shown="No Error" w515 {
                        tunnel: [w533 w535] -> w525
                        tunnel: w524 -> [w533 _]
                        tunnel: w516 -> [_ w535]
                        tunnel: w518 -> [_ w534]
                        frame No Error {
                        }
                        frame Error {
                          n177 = call <instrlib>:"niScope Abort.vi"("instrument handle"=w534) -> ()  [unwired: 13 in, 2 out]
                        }
                      }
                      n178 = Index Array(array=w530) -> (element=w529:T26)  [unwired: 1 in]
                      n179 = Unbundle By Name(w515) -> ("status"=w514:bool)
                      n180 = Unbundle By Name(w529) -> ("gain"=w531:dbl)
                    }
                  }
                  n181 = expression code="x*1000"(w495) -> (w494:dbl)
                  n182 = Bundle("gain"=w507, "wfm"=w506, "Reverse?"=w502, w500, "status"=w497) -> (w503:T27)  [unwired: 1 in]
                  n183 = Enqueue Element(queue=w504, element=w503, timeout in ms (-1)=w494) -> (queue out=w505:refnum<queue>)  [unwired: 1 in, 2 out]
                }
              }
              frame "AlazarTech" {
                # "insert empty array for channel 5.\nThs is for 4 ch card"
                n184 = Bundle By Name(cluster=w540, "DigTimeOut"=4000.0 ("time out")) -> (w538:T8)
                n185 = call "AlazarStackChannels5Pass.vi"("lines per plane"=w543, "AlazarCluster"=w544, "Digitizer Settings"=w538, "Channels"=4 ("dimension size"), "Extra Shift"=w545) -> ("Voltage Scale"=w542:dbl, "Return Code"=w541:u32, "ChStackDataOut"=w536:i16[][][])  [unwired: 3 in, 1 out]
                n186 = Equal?(x=w541, y=u32 579) -> (x = y?=w548:bool)
                n187 = Build Array (concatenate)(w536, w547) -> ()  [unwired: 1 out]
                n188 = call "DelayPtsAdjust.vi"("Digitizer Settings"=w538) -> ("PostDelayCorrection"=w537:u32)  [unwired: 9 in, 1 out]
                n189 = for {
                  tunnel: w553 -> [w555]
                  tunnel: [w566] -> w552
                  tunnel: w551 -> [w565]
                  tunnel: w542 -> [w563]
                  tunnel: w543 -> [w561]
                  tunnel: w536 -> [w560] mode=indexing
                  tunnel: w550 -> [w559]
                  tunnel: w548 -> [w557]
                  tunnel: w537 -> [w554]
                  i -> [w562]
                  n190 = case shown="0, Default" w562 {
                    tunnel: [w571 i16[][] [[1]]] -> w558
                    tunnel: w561 -> [w569 _]
                    tunnel: w560 -> [w568 _]
                    tunnel: w559 -> [w570 _]
                    tunnel: w554 -> [w567 _]
                    frame 0, Default {
                      n191 = Array Subset(array=w568, length (row)=w569, index (col)=w567, length (col)=w570) -> (w571:i16[][])  [unwired: 1 in]
                    }
                    frame 6 {
                    }
                  }
                  n192 = Bundle("Voltage Scale"=w563, w558, "Reverse?"=w565, w562, w557) -> (w564:T28)  [unwired: 1 in]
                  n193 = Enqueue Element(queue=w555, element=w564, timeout in ms (-1)=20.0 ("time out")) -> (queue out=w566:refnum<queue>)  [unwired: 1 in, 2 out]
                }
              }
              frame "LeCroy" {
                # "insert empty array for channel 5.\nThs is for 4 ch card"
                n194 = Bundle By Name(cluster=w579, "DigTimeOut"=4000.0 ("time out")) -> (w577:T8)
                n195 = for {
                  N: 5 ("dimension size") -> [_]
                  tunnel: w584 -> [w591]
                  tunnel: [w598] -> w583
                  tunnel: w582 -> [w597]
                  tunnel: w580 -> [w595]
                  tunnel: w581 -> [w594]
                  tunnel: w577 -> [w588]
                  tunnel: w575 -> [w590]
                  tunnel: TRUE ("x = y?") -> [w589]
                  tunnel: w573 -> [w585] mode=indexing
                  i -> [w586]
                  n196 = case shown="True" w585 {
                    tunnel: [w605 w606] -> w593
                    tunnel: w595 -> [_ _]
                    tunnel: w594 -> [w604 _]
                    tunnel: w590 -> [_ w606]
                    tunnel: w588 -> [w603 _]
                    tunnel: [w600 _] -> w587
                    tunnel: w586 -> [w599 _]
                    frame True {
                      n197 = call "GetAcqSeqLeCroy.vi"("Digitizer Settings"=w603, "Source (0: Channel 1)"=w599, "save?"=FALSE) -> ("Raw VGain (scale)"=w600:dbl, "Data Array"=w602:i16[][])  [unwired: 18 in, 5 out]
                      n198 = Array Subset(array=w602, length (col)=w604) -> (w605:i16[][])  [unwired: 3 in]
                    }
                    frame False {
                    }
                  }
                  n199 = Bundle("Raw VGain (scale)"=w587, w593, "Reverse?"=w597, w586, "x = y?"=w589) -> (w596:T29)  [unwired: 1 in]
                  n200 = Enqueue Element(queue=w591, element=w596, timeout in ms (-1)=20.0 ("time out")) -> (queue out=w598:refnum<queue>)  [unwired: 1 in, 2 out]
                }
              }
            }
          }
          frame #2 {
            n201 = Wait on Notification(notifier=w608, timeout in ms (-1)=5) -> (timed out?=w609:bool)  [unwired: 2 in, 3 out]
            n202 = Not(x=w609) -> (.not. x?=w607:bool)
          }
          frame #3 {
            n203 = case shown="\"AlazarTech\"" w614 {
              tunnel: w612 -> [_ w617]
              tunnel: w611 -> [_ w616]
              tunnel: w613 -> [_ w615]
              frame "Acqiris Digitizer", Default {
              }
              frame "AlazarTech" {
                n204 = case shown="512, Default" w615 {
                  tunnel: w617 -> [_ w631]
                  tunnel: w616 -> [_ w630]
                  frame 0 {
                  }
                  frame 512, Default {
                    w618 = u32 268435538 items=["Data Width"=268435465, "Set/Get Async BuffSize"=268435513, "Set/Get Async Buffcount"=268435520, "Get Data Format"=268435522, "Get Samples Per Timestamp Clock"=268435524, "Get Records Captured"=268435525, "Get Async Buffers Pending"=268435536, "Get Async Buffers Pending Full"=268435537, "Get Async Buffers Pending Empty"=268435538, "ECC Mode"=268435528, "Get Aux Input Level"=268435529, "Get Channels Per Board"=268435568, "Pack Mode"=268435570, "Get FPGA Temperature"=268435584] ("Parameter")
                    w619 = u32 268435537 items=["Data Width"=268435465, "Set/Get Async BuffSize"=268435513, "Set/Get Async Buffcount"=268435520, "Get Data Format"=268435522, "Get Samples Per Timestamp Clock"=268435524, "Get Records Captured"=268435525, "Get Async Buffers Pending"=268435536, "Get Async Buffers Pending Full"=268435537, "Get Async Buffers Pending Empty"=268435538, "ECC Mode"=268435528, "Get Aux Input Level"=268435529, "Get Channels Per Board"=268435568, "Pack Mode"=268435570, "Get FPGA Temperature"=268435584] ("Parameter")
                    w627 = u32 268435536 items=["Data Width"=268435465, "Set/Get Async BuffSize"=268435513, "Set/Get Async Buffcount"=268435520, "Get Data Format"=268435522, "Get Samples Per Timestamp Clock"=268435524, "Get Records Captured"=268435525, "Get Async Buffers Pending"=268435536, "Get Async Buffers Pending Full"=268435537, "Get Async Buffers Pending Empty"=268435538, "ECC Mode"=268435528, "Get Aux Input Level"=268435529, "Get Channels Per Board"=268435568, "Pack Mode"=268435570, "Get FPGA Temperature"=268435584] ("Parameter")
                    n205 = Unbundle By Name(w630) -> ("Digitizer ID Cluster.Acqiris/Alazar/SP ID"=w629:u32[])
                    n206 = Index Array(array=w629) -> (element=w628:u32)  [unwired: 1 in]
                    n207 = call "AlazarGetParameter.vi"("Parameter"=w627, "Handle"=w628) -> ("error out"=w623:errorcluster, "Handle"=w626:u64)  [unwired: 2 in, 2 out]
                    n208 = call "AlazarGetParameter.vi"("error in (no error)"=w623, "Parameter"=w618, "Handle"=w626) -> ("error out"=w622:errorcluster, "Handle"=w625:u64)  [unwired: 1 in, 2 out]
                    n209 = call "AlazarGetParameter.vi"("error in (no error)"=w622, "Parameter"=w619, "Handle"=w625) -> ("error out"=w621:errorcluster, "Value"=w620:i32, "Handle"=w624:u64)  [unwired: 1 in, 1 out]
                    n210 = case shown="2, Default" w620 {
                      selector: w620 -> [_ w636]
                      tunnel: w631 -> [_ w638]
                      tunnel: w624 -> [_ w633]
                      tunnel: w621 -> [_ w632]
                      frame 0, 1 {
                      }
                      frame 2, Default {
                        # "Delete surplus buffers"
                        n211 = Decrement(x=w636) -> (x-1=w634:i32)
                        n212 = Unbundle(w638) -> ("data value reference"=w637:refnum<data-value>)  [unwired: 2 out]
                        n213 = for {
                          N: w634 -> [_]
                          tunnel: w637 -> [w641]
                          tunnel: u32 1 ("uTimeout_ms") -> [w642]
                          tunnel: w633 -> [w640]
                          tunnel: w632 -> [w639]
                          n214 = in-place {
                            in-place-border: w642 -> [w645]
                            in-place-border: w640 -> [w644]
                            in-place-border: w639 -> [w643]
                            n215 = in-place-dvr #3(w641) -> (w646:u16[])  [unwired: 1 out]
                            n216 = call "AlazarWaitNextAsyncBufferCompleteU16.vi"("error in (no error)"=w643, "Timeout (ms)"=w645, "Buffer"=w646, "Handle"=w644) -> ("Buffer"=w647:u16[])  [unwired: 3 out]
                            n217 = in-place-dvr #3(w647) -> ()  [unwired: 2 out]
                          }
                        }
                      }
                    }
                  }
                }
              }
            }
          }
          frame #4 {
            # "Check if motion program is paused at end of run. Rare case of done may come up."
            n218 = case shown="4" 0 {
              tunnel: w648 -> [_ w651]
              frame 0, Default {
              }
              frame 4 {
                n219 = Unbundle By Name(w651) -> ("Motion System"=w650:T5)
                n220 = case shown="\"NI 735x\"" w650 {
                  tunnel: w651 -> [_ w652]
                  frame "MM3000", Default {
                  }
                  frame "NI 735x" {
                    n221 = disable-structure shown="Disabled" {
                      disable-tunnel: w652 -> [w654 _]
                      frame Disabled {
                        n222 = Unbundle By Name(w654) -> ("Motion Bd ID"=w653:u8)
                        n223 = while {
                          tunnel: [w666] -> _
                          tunnel: [w662] -> _
                          tunnel: enum16{"Done", "Playing", "Paused", "Storing"}."Paused" ("Program Status") -> [w665]
                          tunnel: w653 -> [w664]
                          tunnel: [w658] -> _
                          tunnel: [30 ("DeviceIn")] -> w655
                          i -> [w658]
                          stop <- w659 stop-if-true
                          n224 = call <vilib>:"Read Program Status.flx"("Program (1)"=T20 8, "Board Id"=w664) -> ("error out"=w662:errorcluster, "Bd Id Out"=w666:T30, "Program Status"=w663:enum16{"Done", "Playing", "Paused", "Storing"})  [unwired: 4 in, 1 out]
                          n225 = Unbundle(w662) -> ("status"=w661:bool)  [unwired: 2 out]
                          n226 = Equal?(x=w665, y=w663) -> (x = y?=w660:bool)
                          n227 = Or(x=w660, y=w661) -> (x .or. y?=w659:bool)
                        }
                        n228 = Wait (ms)(milliseconds to wait=w655) -> ()  [unwired: 1 out]
                      }
                      frame Enabled {
                      }
                    }
                  }
                }
              }
            }
          }
        }
      }
      n229 = Release Queue(queue=w278, force destroy? (F)=w271) -> ()  [unwired: 1 in, 3 out]
      n230 = Delete Data Value Reference(data value reference=w277) -> ()  [unwired: 1 in, 2 out]
    }
    frame #5 {
      n231 = Unbundle By Name(w668) -> ("Motion System"=w671:T5, "Motion Bd ID"=w670:u8)
      n232 = Unbundle By Name(w674) -> ("Main Digitizer"=w673:T9, "Dig Config"=w672:T10)
      n233 = case shown="\"NI 735x\"" w671 {
        tunnel: w676 -> [w681 _]
        tunnel: w670 -> [w680 _]
        frame "NI 735x" {
          n234 = disable-structure shown="Disabled" {
            disable-tunnel: w681 -> [w683 _]
            disable-tunnel: w680 -> [w682 _]
            frame Disabled {
              n235 = call <vilib>:"Enable Breakpoint Output.flx"("Enable Breakpoint"=FALSE, "Axis or Encoder"=w683, "Board ID"=w682) -> ()  [unwired: 1 in, 6 out]
            }
            frame Enabled {
            }
          }
        }
        frame "No Motion Card", Default {
        }
      }
      n236 = case shown="\"AlazarTech\"" w673 {
        tunnel: w674 -> [w686 _ w691]
        tunnel: w675 -> [_ _ w689]
        frame "Acqiris Digitizer" {
          n237 = Unbundle By Name(w686) -> ("Digitizer ID Cluster.NI Instr Handles"=w685:refnum<k15>[])
          n238 = for {
            tunnel: w685 -> [w687] mode=indexing
            n239 = call <instrlib>:"niScope Abort.vi"("instrument handle"=w687) -> ()  [unwired: 13 in, 2 out]
          }
        }
        frame "LeCroy", Default {
        }
        frame "AlazarTech" {
          n240 = Unbundle By Name(w691) -> ("Digitizer ID Cluster.Acqiris/Alazar/SP ID"=w690:u32[])
          n241 = Unbundle By Name(w689) -> ("data value reference"=w688:refnum<data-value>)
          n242 = for {
            tunnel: w690 -> [w693] mode=indexing
            n243 = call "AlazarAbortAsyncRead.vi"("Handle"=w693) -> ("Handle"=w695:u64, "error out"=w694:errorcluster)  [unwired: 1 in, 1 out]
            n244 = call "AlazarConfigureAuxIO.vi"("error in (no error)"=w694, "Mode"=u32 13, "Handle"=w695) -> ()  [unwired: 1 in, 3 out]
          }
          n245 = Delete Data Value Reference(data value reference=w688) -> ()  [unwired: 1 in, 2 out]
        }
      }
      n246 = Cancel Notification(0:w677) -> ()  [unwired: 1 in, 3 out]
      n247 = case shown="\"Hawaii\", Default" w678 {
        tunnel: w668 -> [w701 _]
        frame "Hawaii", Default {
          w702 = u16 1 items=["Function Gen Input", "Motion Trig", "Internal RT Motion Trig", "Internal CTR 1 Output"] ("Trig Source")
          n248 = Unbundle By Name(w701) -> ("GL Ref Out"=w700:refnum<k7>)
          n249 = call "RouteTrigSource.vi"("Galil.IGalil"=w700, "Trig Source"=w702) -> ()  [unwired: 9 in, 1 out]
        }
        frame "UHI Allen", "CUMC RT" {
        }
      }
      n250 = case shown="\"5-CH pulser w/ ann array\"" w672 {
        tunnel: w679 -> [_ w696]
        frame "Single channel", Default {
        }
        frame "5-CH pulser w/ ann array" {
          n251 = for {
            tunnel: w696 -> [w699] mode=indexing
            n252 = call <vilib>:"DAQmx Stop Task.vi"("task/channels in"=w699) -> ("task out"=w698:refnum<k21>, "error out"=w697:errorcluster)  [unwired: 13 in]
            n253 = call <vilib>:"DAQmx Clear Task.vi"("task in"=w698, "error in"=w697) -> ()  [unwired: 13 in, 1 out]
          }
        }
      }
      n254 = Unbundle By Name(w668) -> ("Motion System"=w669:T5)
    }
  }
  n255 = case shown="\"NI 735x\"" w8 {
    tunnel: w28 -> [w704 w754 _]
    tunnel: w27 -> [w709 _ _]
    tunnel: w26 -> [w708 w736 _]
    tunnel: w25 -> [w707 w753 _]
    tunnel: w7 -> [w703 w757 _]
    frame "NI 735x" {
      # "Return to start location and reset to original value"
      n256 = disable-structure shown="Disabled" {
        disable-tunnel: w709 -> [w732 _]
        disable-tunnel: w708 -> [w731 w733]
        disable-tunnel: w707 -> [w730 _]
        disable-tunnel: [w729 w733] -> w706
        disable-tunnel: [w726 _] -> w705
        disable-tunnel: w704 -> [w715 _]
        disable-tunnel: w703 -> [w711 _]
        frame Disabled {
          n257 = Unbundle By Name(w711) -> ("Motor Parameters.velocity ct/s"=w717:dbl[], "Motor Parameters.accel ct/s^2"=w716:dbl[], "Motion Bd ID"=w710:u8)
          n258 = call-poly <vilib>:"Wait for Move Complete.flx"("error in (no error)"=w731, "Board ID"=w710) -> ("error out"=w718:errorcluster, "Bd ID Out"=w719:T30)  [unwired: 6 in, 2 out]
          n259 = call <vilib>:"Stop Program.flx"("error in (no error)"=w718, "Program (1)"=w732, "Board ID"=w719) -> ("error out"=w727:errorcluster, "Bd ID Out"=w728:T30)  [unwired: 4 out]
          n260 = Decrement(x=w715) -> (x-1=w714:u16)
          n261 = call "MoveMotor.vi"("error in (no error)"=w727, "Target Position (0)"=w730, "Axis or Vector Space"=w715, "Motion Bd ID"=w728) -> ("error out"=w721:errorcluster, "Resource Output"=w720:u16, "Bd ID Out"=w722:u8)  [unwired: 5 in]
          n262 = Index Array(array=w717, index=w714) -> (element=w713:dbl)
          n263 = Index Array(array=w716, index=w714) -> (element=w712:dbl)
          n264 = call "Load Acceleration/Deceleration.flx"("Acceleration (100000)"=w712, "error in (no error)"=w721, "Axis or Vector Space"=w720, "Board ID"=w722) -> ("error out"=w725:errorcluster, "Resource Output"=w723:T31, "Bd ID Out"=w724:T30)  [unwired: 1 in, 2 out]
          n265 = call <vilib>:"Load Velocity.flx"("Velocity (10000)"=w713, "error in (no error)"=w725, "Axis or Vector Space"=w723, "Board ID"=w724) -> ("error out"=w729:errorcluster, "Bd ID Out"=w726:T30)  [unwired: 4 out]
        }
        frame Enabled {
        }
      }
      "error out" <- w706
      "Bd ID Out" <- w705
    }
    frame "Galil" {
      # "Return to start location and reset to original value"
      n266 = Unbundle By Name(w757) -> ("Motor Parameters.velocity ct/s"=w767:dbl[], "Motor Parameters.accel ct/s^2"=w766:dbl[], "GL Ref Out"=w739:refnum<k7>)
      n267 = call "GL Command Set.vi"("Command"=Command_Menu."Halt Execute", "error in (no error)"=w736, "Value"=-1, "Galil.IGalil"=w739) -> ("error out"=w737:errorcluster, "ref out"=w738:refnum<k7>)  [unwired: 3 in, 3 out]
      n268 = Decrement(x=w754) -> (x-1=w744:u16)
      n269 = call "GL Command Set.vi"("Command"=Command_Menu."BreakPoint", "error in (no error)"=w737, "Value"=0, "Axis"=w744, "Galil.IGalil"=w738) -> ("error out"=w749:errorcluster, "Axis Out"=w745:T32, "ref out"=w750:refnum<k7>)  [unwired: 2 in, 2 out]
      n270 = Index Array(array=w767, index=w744) -> (element=w756:dbl)
      n271 = Index Array(array=w766, index=w744) -> (element=w755:dbl)
      n272 = call "GL CheckForMotion.vi"("error in"=w749, "Axis"=w745, "Refnum in"=w750) -> ("error out"=w747:errorcluster, "Axis out"=w746:T32, "Refnum out"=w748:refnum<k7>)  [unwired: 6 in]
      n273 = call "GL Set Operation Mode.vi"("position cts (abs/rel)"=w753, "error in (no error)"=w747, "Axis"=w746, "Galil.IGalil"=w748) -> ("error out"=w740:errorcluster, "Axis Out Output"=w752:T32, "Galil Out"=w751:refnum<k7>)  [unwired: 5 in]
      n274 = call "GL Command Set.vi"("Command"=Command_Menu."Velocity", "error in (no error)"=w740, "Value"=w756, "Axis"=w752, "Galil.IGalil"=w751) -> ("error out"=w764:errorcluster, "Axis Out"=w761:T32, "ref out"=w765:refnum<k7>)  [unwired: 2 in, 2 out]
      n275 = call "GL Command Set.vi"("Command"=Command_Menu."Acceleration", "error in (no error)"=w764, "Value"=w755, "Axis"=w761, "Galil.IGalil"=w765) -> ("error out"=w762:errorcluster, "Axis Out"=w760:T32, "ref out"=w763:refnum<k7>)  [unwired: 2 in, 2 out]
      n276 = call "GL Command Set.vi"("Command"=Command_Menu."Deceleration", "error in (no error)"=w762, "Value"=w755, "Axis"=w760, "Galil.IGalil"=w763) -> ()  [unwired: 2 in, 5 out]
    }
    frame "No Motion Card", Default {
    }
  }
